vi "External Actuators Fudge.vi"(9 "Load\nCells":dbl[](array[numeric])=[-0.033, -0.464, -0.305, -0.519, -0.312, 0.351], 11 "LVDTs":dbl[](array[numeric])=[0.129, -0.195, 0.192, 0.128, -0.193, 1.235002]) -> (2 "Actuators Out":dbl[](array[numeric]))   [LabVIEW 2009]
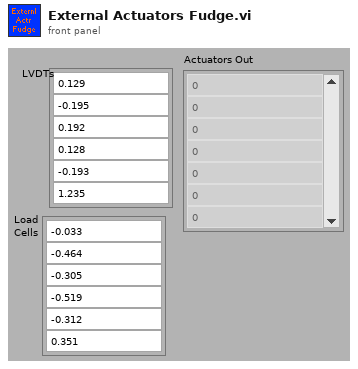
[diagram p1: front panel]
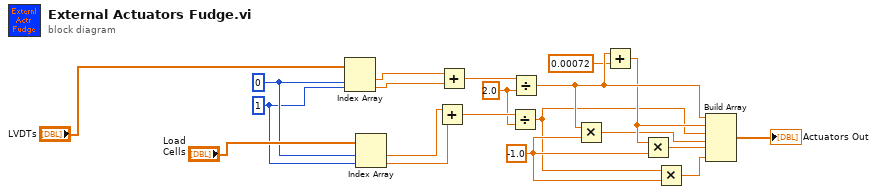
[diagram p0: block diagram]
diagram:
  w10 = -1.0 ("y")
  w16 = 2.0 ("y")
  w3 = 1 ("index")
  w4 = 0 ("index")
  n1 = Index Array(array="LVDTs", index #1=w4, index #2=w3) -> (element #1=w20:dbl, element #2=w19:dbl)
  n2 = Index Array(array="Load\nCells", index #1=w4, index #2=w3) -> (element #1=w2:dbl, element #2=w1:dbl)
  n3 = Add(x=w2, y=w1) -> (x+y=w17:dbl)
  n4 = Add(x=w20, y=w19) -> (x+y=w18:dbl)
  n5 = Divide(x=w17, y=w16) -> (x/y=w8:dbl)
  n6 = Divide(x=w18, y=w16) -> (x/y=w15:dbl)
  n7 = Multiply(x=w15, y=w10) -> (x*y=w11:dbl)
  n8 = Add(x=w15, y=0.00072) -> (x+y=w13:dbl)
  n9 = Multiply(x=w13, y=w10) -> (x*y=w12:dbl)
  n10 = Multiply(x=w8, y=w10) -> (x*y=w9:dbl)
  n11 = Build Array(w15, w13, w8, w11, w12, w9) -> (→"Actuators Out":dbl[])
